vi "CreateSerializationSession.vi"(8 "error in":errorcluster) -> (0 "error out":errorcluster, 3 "Serialization Session ID":T1)   [LabVIEW 2019, in "grpc-lvsupport.lvlib"]
uses:
  grpc-lvsupport.lvlib
  Shared/grpcId.ctl
  <vilib>/Utility/error.llb/Error Cluster From Error Code.vi
  <resource>/labview_grpc_server.dll
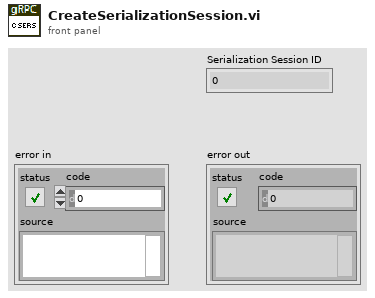
[diagram p1: front panel]
types:
  T1 = typedef "grpc-lvsupport.lvlib/grpcId.ctl" = u64
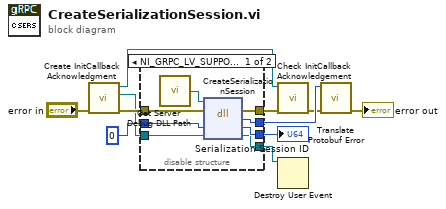
[diagram p0: block diagram]
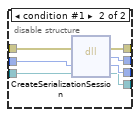
[diagram p2: hidden frame]
diagram:
  n1 = call "Create InitCallback Acknowledgment.vi"("error in (no error)"="error in") -> ("error out"=w5:errorcluster, "Init'd"=w2:refnum<user-event>, "InitCallbackAck Registration"=w3:refnum<event-registration>)  [unwired: 8 in]
  n2 = disable-structure shown="NI_GRPC_LV_SUPPORT_DEBUG==True&&RUN_TIME_ENGINE==False" {
    disable-tunnel: [w19 w26] -> w10
    disable-tunnel: u64 0 ("gRPCId") -> [w17 w25]
    disable-tunnel: [w16 w24] -> w8
    disable-tunnel: [w15 w23] -> w6
    disable-tunnel: w5 -> [w14 w22]
    disable-tunnel: w2 -> [w13 w21]
    disable-tunnel: [w12 w20] -> w1
    frame condition #0 (active) {
      n3 = call "Get Server Debug DLL Path.vi"() -> ("Server Debug DLL Path"=w18:path)
      n4 = dll-call lib="?" fn="CreateSerializationSession"(path in=w18, error in=w14, "serializationId"=w17, "InitCallbackAck"=w13) -> (error out=w19:errorcluster, "return type"=w15:i32, "serializationId"=w16:u64, "InitCallbackAck"=w12:refnum<user-event>)  [unwired: 1 in, 1 out]
    }
    frame condition #1 {
      n5 = dll-call lib="C:/Program Files (x86)/National Instruments/LabVIEW 2024/resource/labview_grpc_server.*" fn="CreateSerializationSession"(error in=w22, "serializationId"=w25, "InitCallbackAck"=w21) -> (error out=w26:errorcluster, "return type"=w23:i32, "serializationId"=w24:u64, "InitCallbackAck"=w20:refnum<user-event>)  [unwired: 2 in, 1 out]
    }
  }
  "Serialization Session ID" <- w8
  n6 = call "Check InitCallback Acknowledgement.vi"("error in (no error)"=w10, "InitCallbackAck Registration"=w3) -> ("error out"=w4:errorcluster)  [unwired: 9 in]
  n7 = Destroy User Event(user event=w1) -> ()  [unwired: 1 in, 1 out]
  n8 = call "Translate Protobuf Error.vi"("error in"=w4, "Error Code"=w6) -> ("error out"=→"error out":errorcluster)  [unwired: 9 in]
